vi "Play Sound File.vi"(8 "error in (no error)":errorcluster, 11 "Sound File":path=path "C:/Users/plane/Dropbox/Research/MTA/DAQ VIs/MTA Shift Toolbox/tng_torpedo_clean.wav") -> (0 "error out":errorcluster)   [LabVIEW 2013]
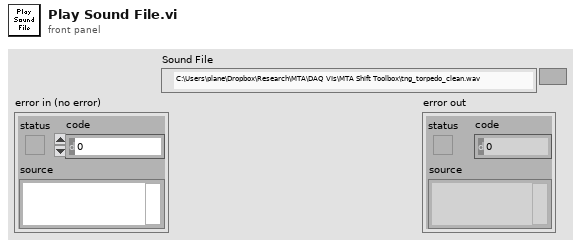
[diagram p1: front panel]
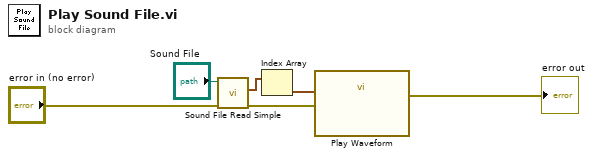
[diagram p0: block diagram]
diagram:
  n1 = call <vilib>:"Sound File Read Simple.vi"("error in (no error)"="error in (no error)", "path"="Sound File") -> ("error out"=w1:errorcluster, "data"=w6:waveform(dbl)[])  [unwired: 6 in, 2 out]
  n2 = Index Array(array=w6) -> (element=w5:waveform(dbl))  [unwired: 1 in]
  n3 = call "Play Waveform"("Data"=w5, "error in"=w1) -> ("error out"=→"error out":errorcluster)  [unwired: 17 in]
